vi "Switch_Heater_on.vi"   [LabVIEW 2016]
uses:
  Global/Global Variables/Data_Display_global.vi
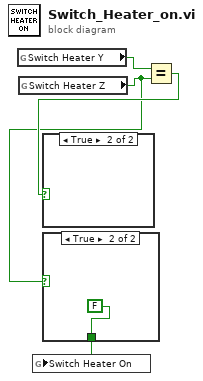
[diagram p0: block diagram]
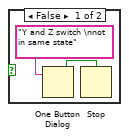
[diagram p2: hidden frame]
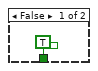
[diagram p3: hidden frame]
diagram:
  n1 = global read "Data_Display_global.vi" "Switch Heater Y"() -> (w3:bool)
  n2 = global read "Data_Display_global.vi" "Switch Heater Z"() -> (w1:bool)
  n3 = case shown="True" w1 {
    tunnel: [TRUE FALSE] -> w4
    frame False {
    }
    frame True {
    }
  }
  n4 = global write "Data_Display_global.vi" "Switch Heater On"(w4) -> ()
  n5 = Equal?(x=w3, y=w1) -> (x = y?=w2:bool)
  n6 = case shown="True" w2 {
    frame False {
      n7 = One Button Dialog(message="Y and Z switch \nnot in same state") -> (true=w7:bool)  [unwired: 1 in]
      n8 = Stop(stop? (T)=w7) -> ()
    }
    frame True {
    }
  }
